vi "Sine.vi"() -> ()   [LabVIEW 2015]
panel:
  out "Waveform Chart 2":dbl(graph)
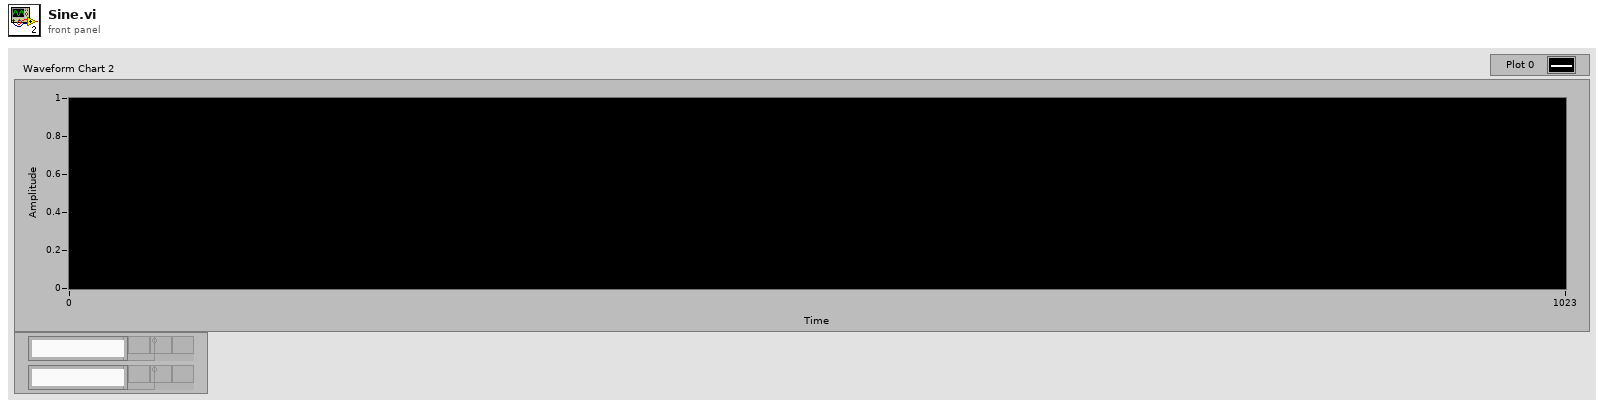
[diagram p1: front panel]
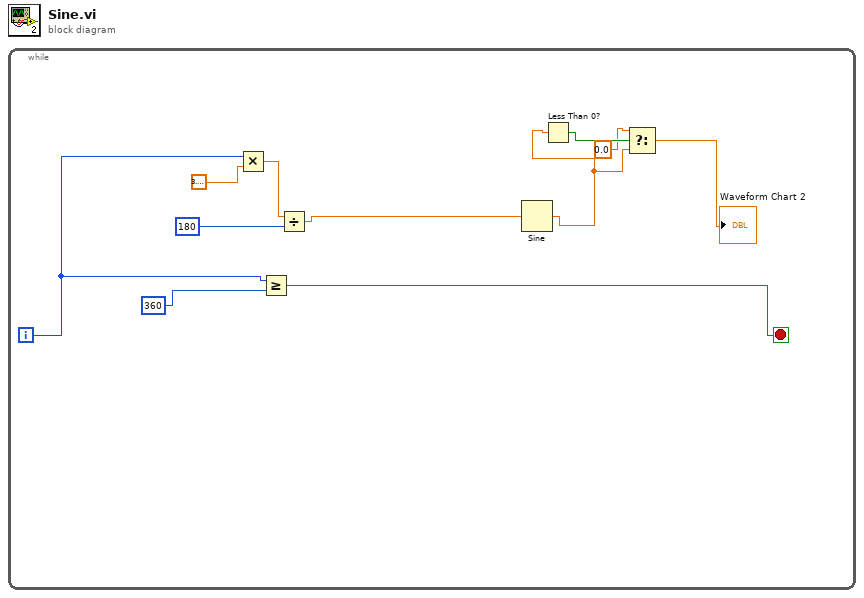
[diagram p0: block diagram]
diagram:
  n1 = while {
    i -> [w8]
    stop <- w5 stop-if-true
    n2 = Multiply(x=w8, y=3.141592653589793) -> (x*y=w9:dbl)
    n3 = Greater Or Equal?(x=w8, y=360) -> (x >= y?=w5:bool)
    n4 = Divide(x=w9, y=180 ("Numeric 3")) -> (x/y=w6:dbl)
    n5 = Sine(x=w6) -> (sin(x)=w2:dbl)
    n6 = Less Than 0?(x=w2) -> (x < 0?=w4:bool)
    n7 = Select(t=0.0 ("f"), s=w4, f=w2) -> (s? t:f=→"Waveform Chart 2":dbl)
  }
